vi "DOOR_ASSIGN.vi"(8 "error In":errorcluster) -> (0 "error out":errorcluster)   [LabVIEW 2017]
uses:
  Controls/Ass. Loop Control.ctl
  <vilib>/Utility/error.llb/DialogType.ctl
  <vilib>/Utility/file.llb/Read Delimited Spreadsheet (string).vi
  <vilib>/Utility/file.llb/Write Delimited Spreadsheet (string).vi
  <vilib>/Utility/config.llb/NI_LVConfig.lvlib
panel:
  in  "REMOVE PART":bool
  in  "ADD PART":bool
  in  "LIST OF PARTS":string(combo)
  in  "DOORS":string(combo)
  in  "DOORS":enum32{"ADD PARTS", "Page 1", "Page 2"}(tab)
  in  "ADDED PART LIST":string(combo)
  in  "REMOVE PART FROM LIST":bool
  in  "ADD PART IN LIST":bool
  in  "NEW PARTS BARCODE":string
  out "DOOR 1":string[](array[string])
  out "DOOR 2":string[](array[string])
  out "DOOR 3":string[](array[string])
  out "DOOR 4":string[](array[string])
  out "DOOR 5":string[](array[string])
  out "DOOR 16":string[](array[string])
  out "DOOR 11":string[](array[string])
  out "DOOR 12":string[](array[string])
  out "DOOR 13":string[](array[string])
  out "DOOR 14":string[](array[string])
  out "DOOR 15":string[](array[string])
  out "USER:-":string
  in  "Stop":bool
  out "DATE/TIME":string
  out "Screen Name":string
  # "Nm"
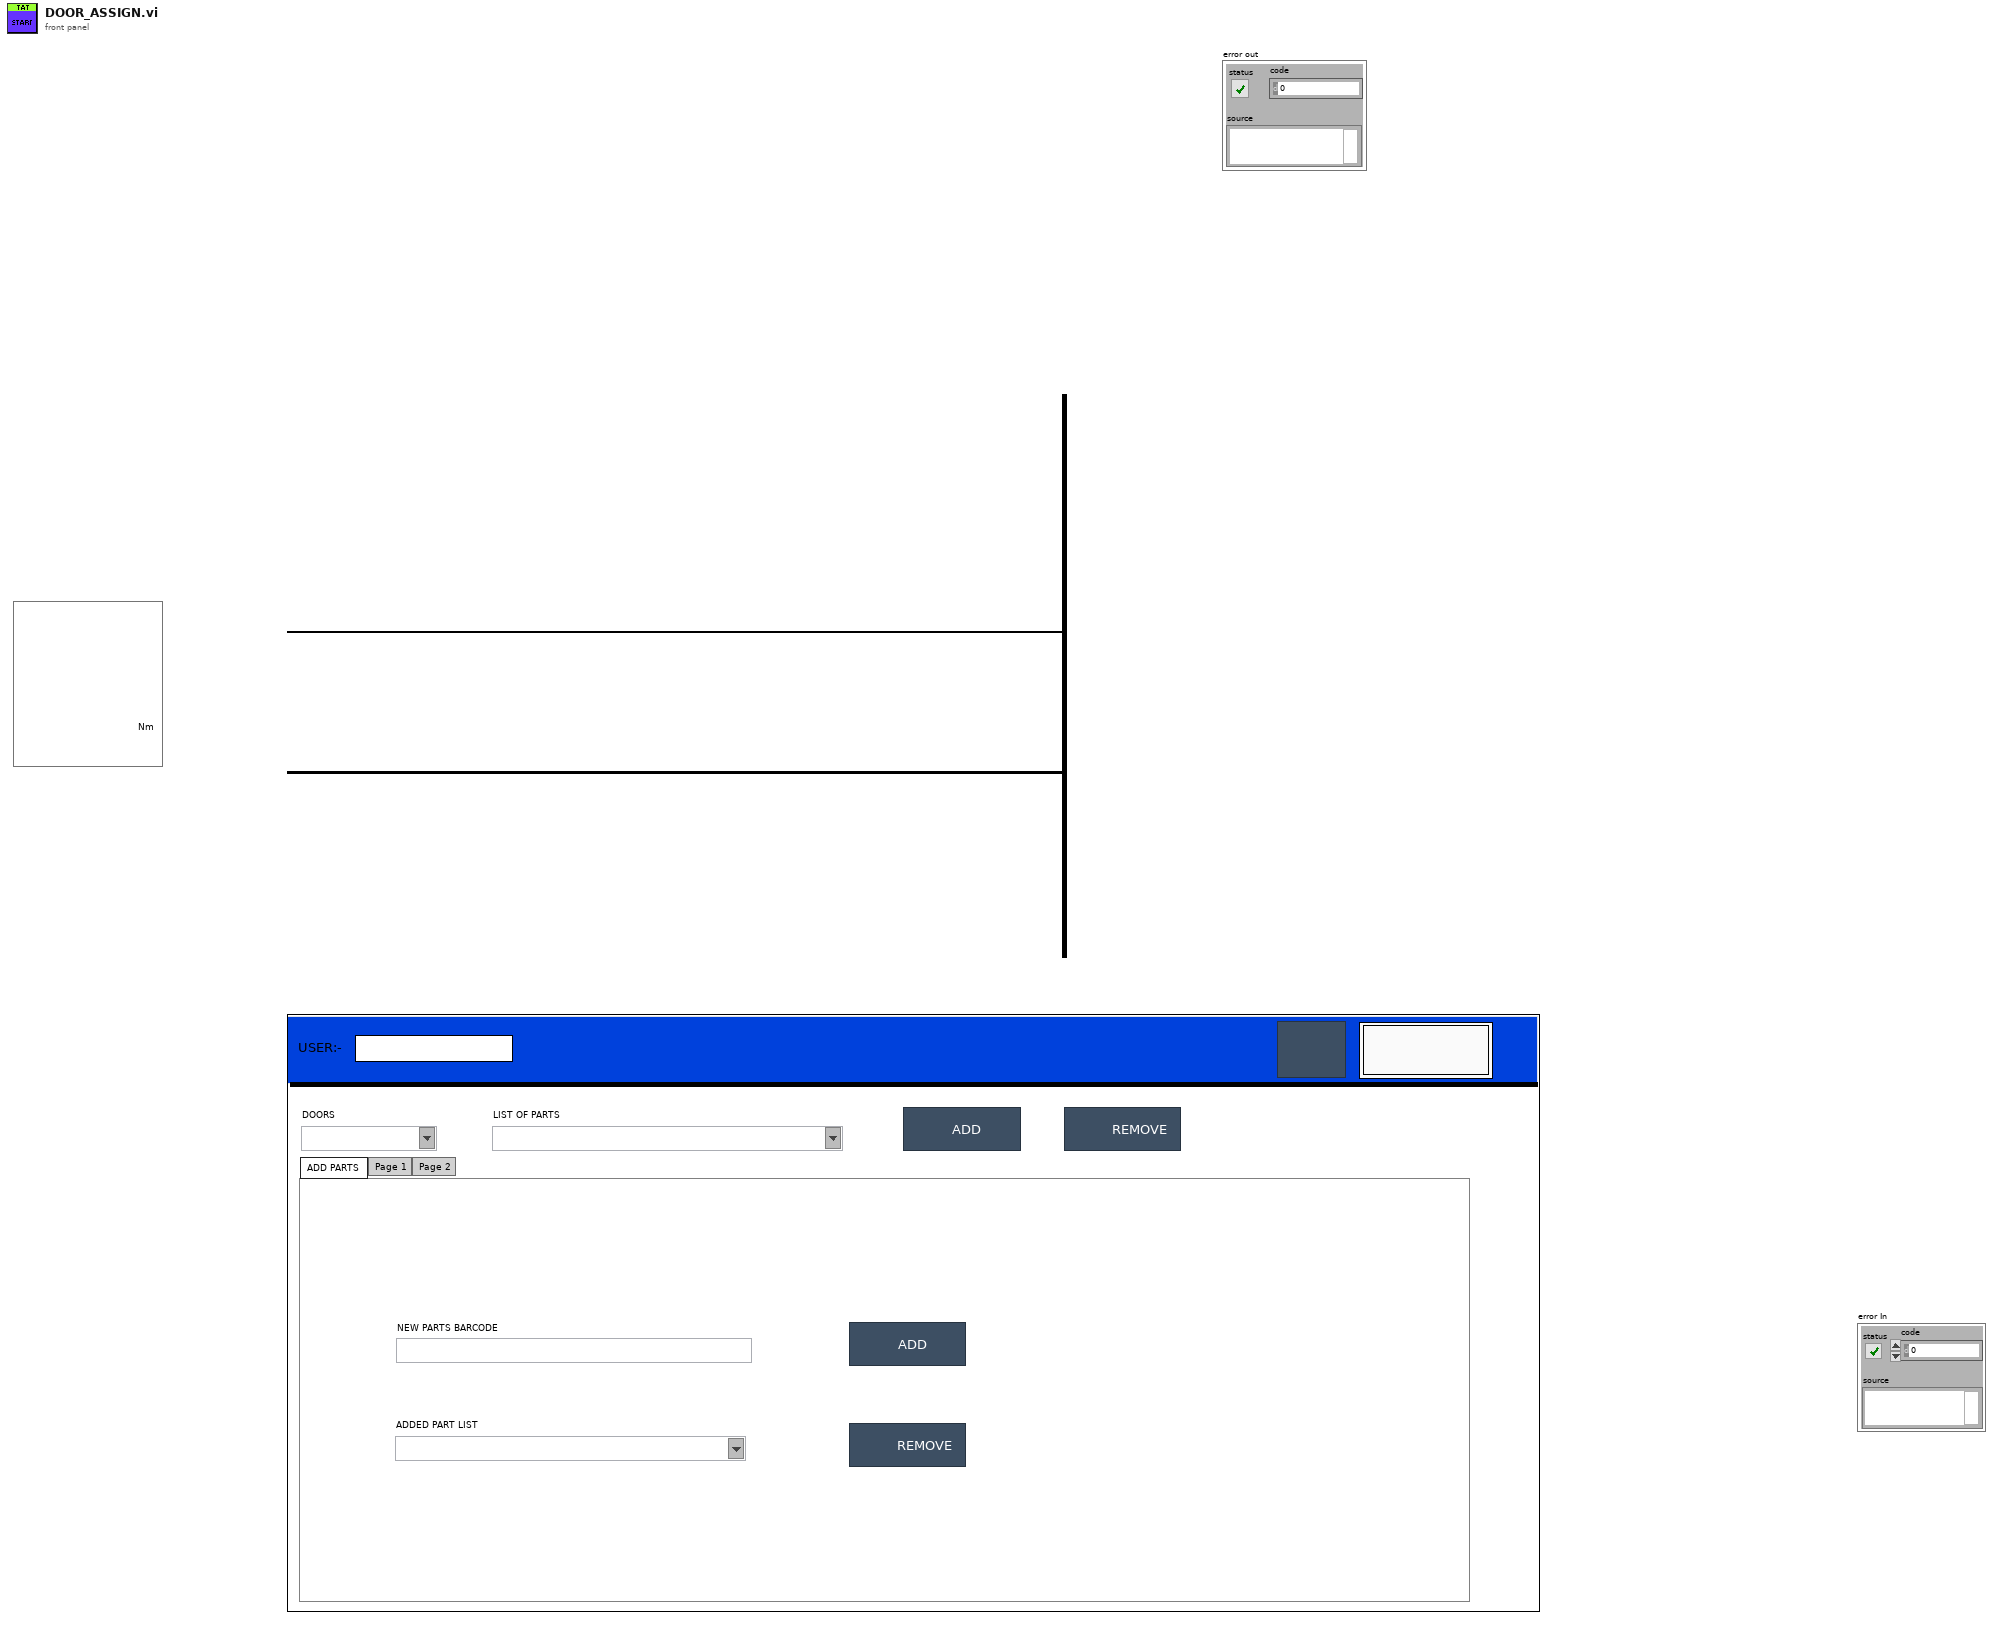
[diagram p1: front panel]
types:
  T1 = cluster{"DOOR ASSIGN":path, "PART LIST":path, "DOOR PART ASSIGN":cluster{"DOOR 1":cluster{"DOOR 1":string[]}, "DOOR 2":cluster{"DOOR 2":string[]}, "DOOR 3":cluster{"DOOR 3":string[]}, "DOOR 4":cluster{"DOOR 4":string[]}, "DOOR 5":cluster{"DOOR 5":string[]}, "DOOR 11":cluster{"DOOR 11":string[]}, "DOOR 12":cluster{"DOOR 12":string[]}, "DOOR 13":cluster{"DOOR 13":string[]}, "DOOR 14":cluster{"DOOR 14":string[]}, "DOOR 15":cluster{"DOOR 15":string[]}, "DOOR 16":cluster{"DOOR 16":string[]}}}
  T2 = typedef "DialogType.ctl" = u16
  T3 = typedef "Ass. Loop Control.ctl" = enum16{"Package_Qty_Count", "GENERATE_QR_PRNT", "Cluster_update", "Waiting_for_scan", "barcode CHECK", "Int", "SaveReport ", "Barcode Print", "Start Cycle", "Wait", "Cycle End", "Stop"}
  T4 = enum32{"invalid app kind", "Development System", "Run Time System", "Student Edition", "Embedded LabVIEW", "Evaluation", "Custom"}
  T5 = cluster{"DOOR 1":string[], "DOOR 2":string[], "DOOR 3":string[], "DOOR 4":string[], "DOOR 5":string[], "DOOR 11":string[], "DOOR 12":string[], "DOOR 13":string[], "DOOR 14":string[], "DOOR 15":string[], "DOOR 16":string[]}
  T6 = typedef "LVComboBoxStrsAndValuesArrayTypeDef.ctl" = cluster{"String":string, "Value":string}[]
  T7 = typedef "NI_LVConfig.lvlib/Config Data RefNum.ctl" = refnum<k1>
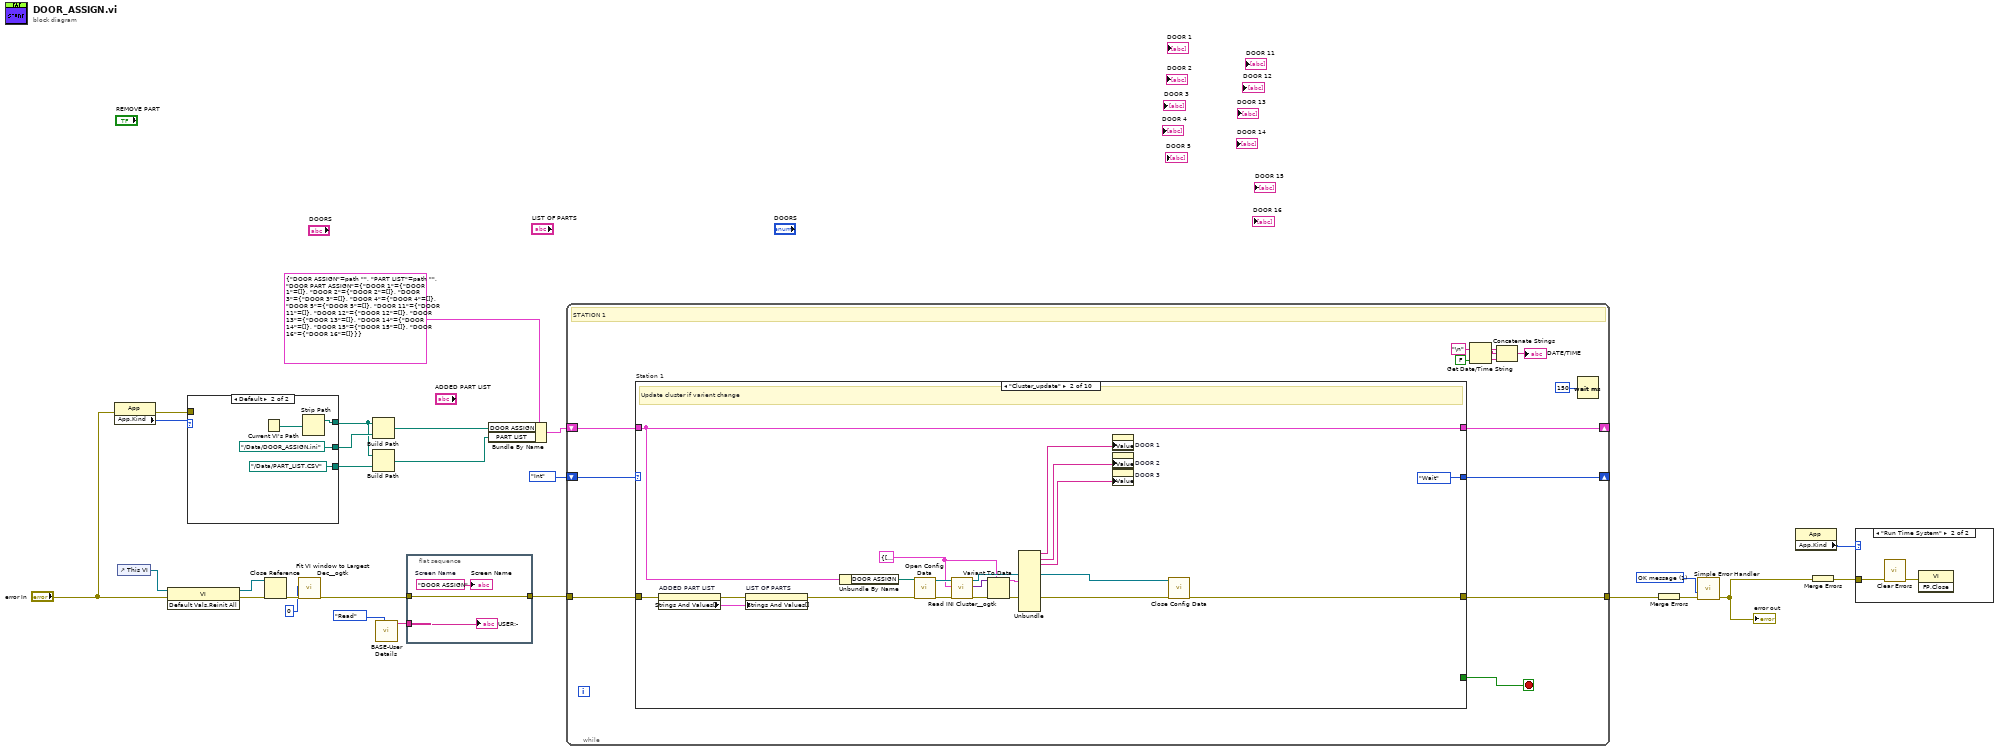
[diagram p0: block diagram]
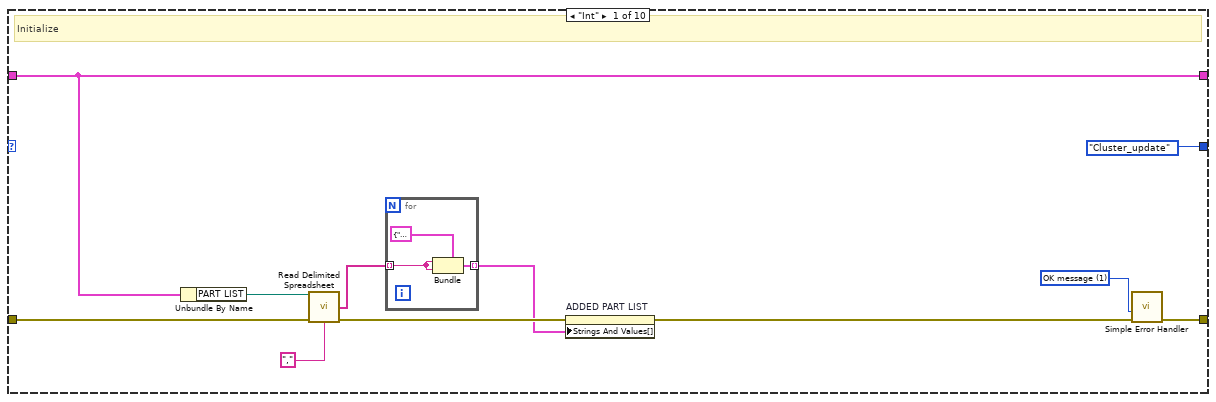
[diagram p3: hidden frame]
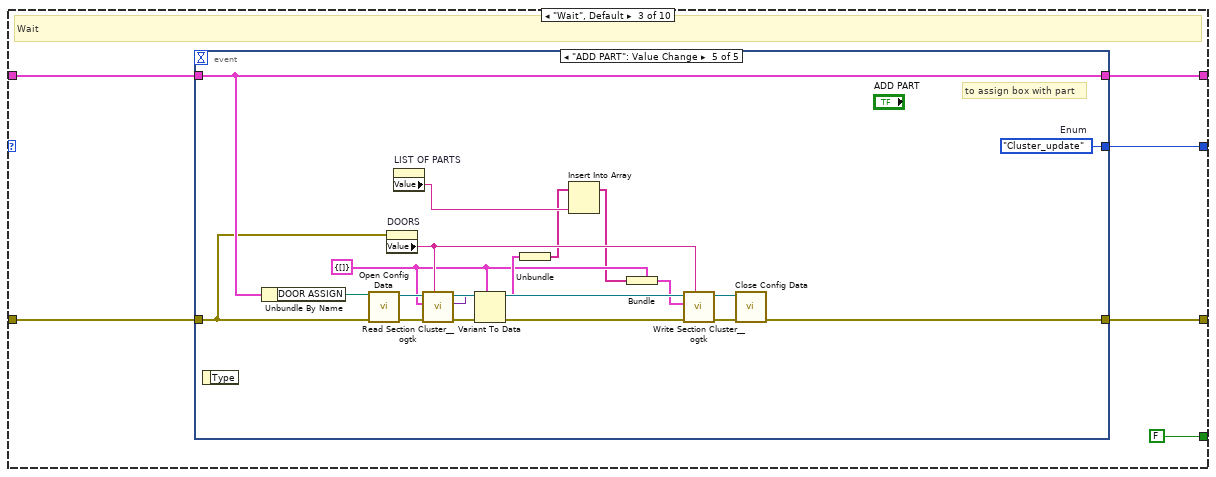
[diagram p4: hidden frame]
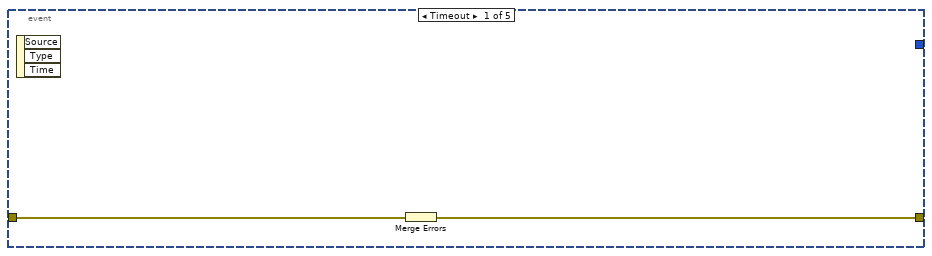
[diagram p5: hidden frame]
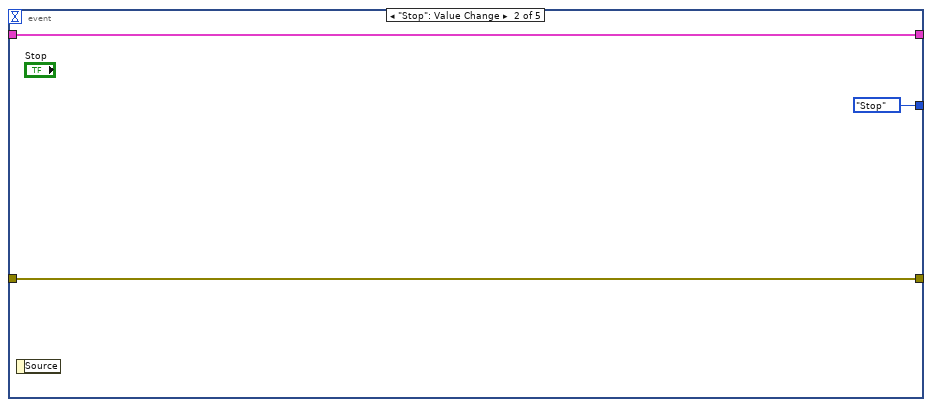
[diagram p6: hidden frame]
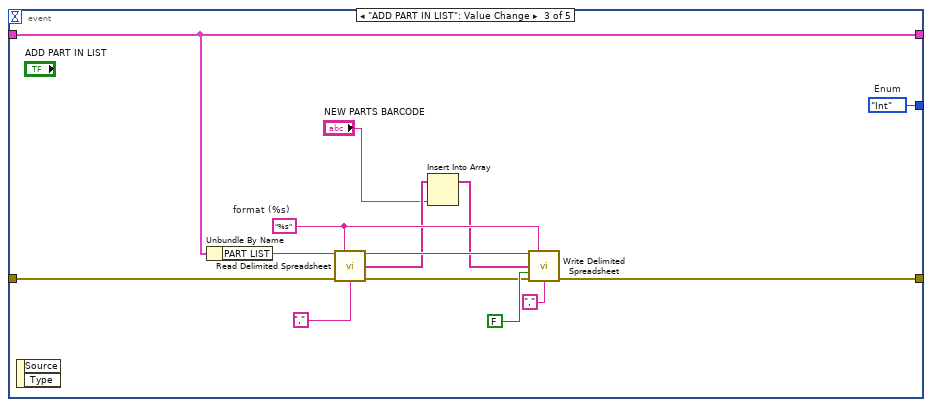
[diagram p7: hidden frame]
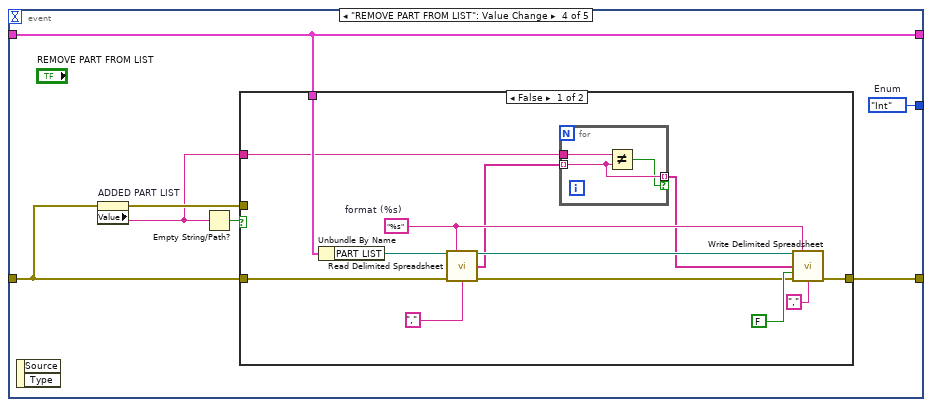
[diagram p8: hidden frame]
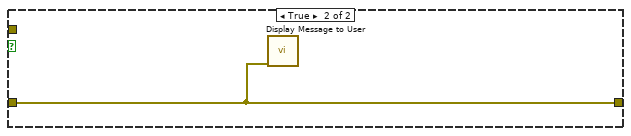
[diagram p9: hidden frame]
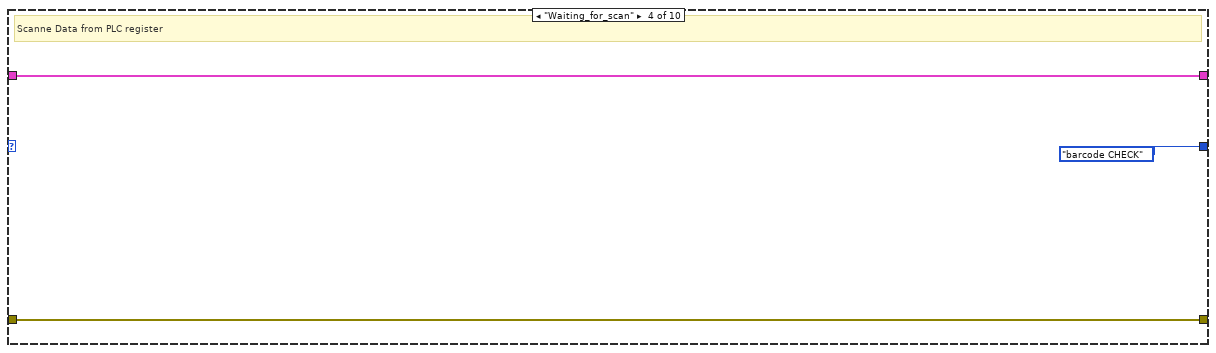
[diagram p10: hidden frame]
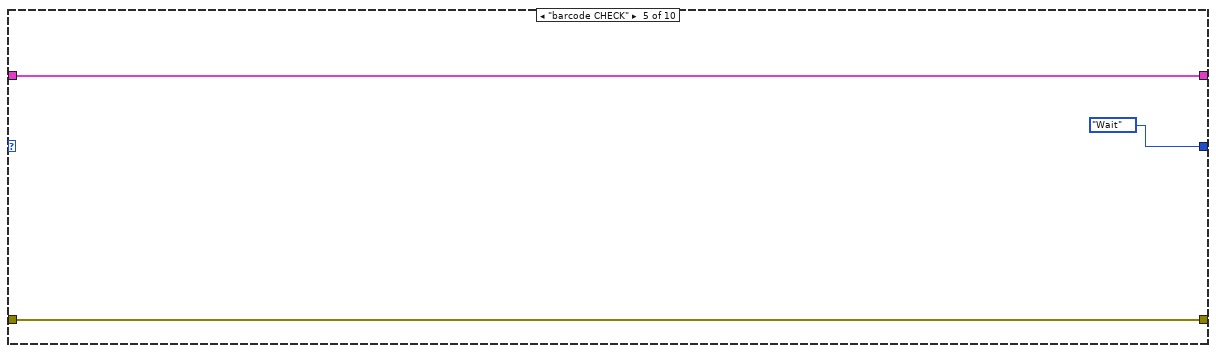
[diagram p11: hidden frame]
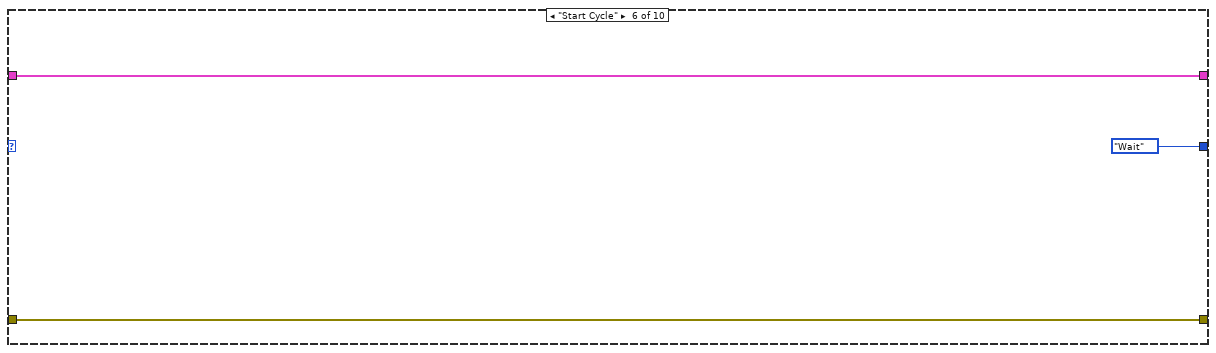
[diagram p12: hidden frame]
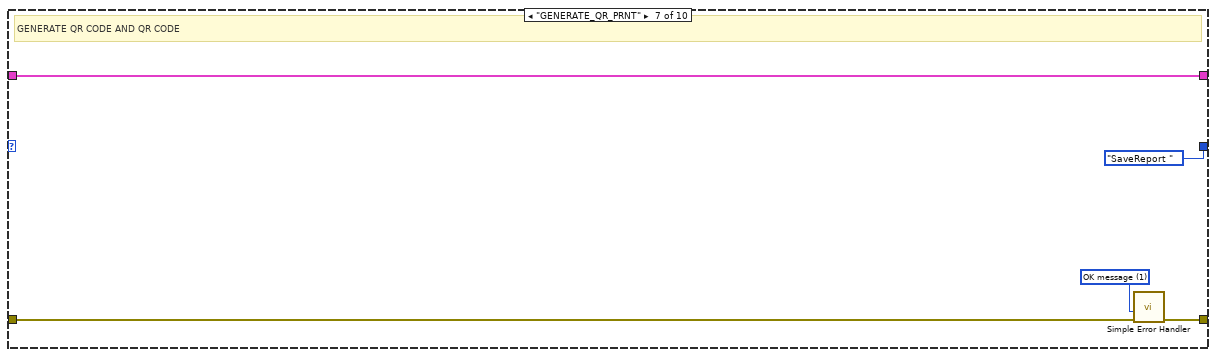
[diagram p13: hidden frame]
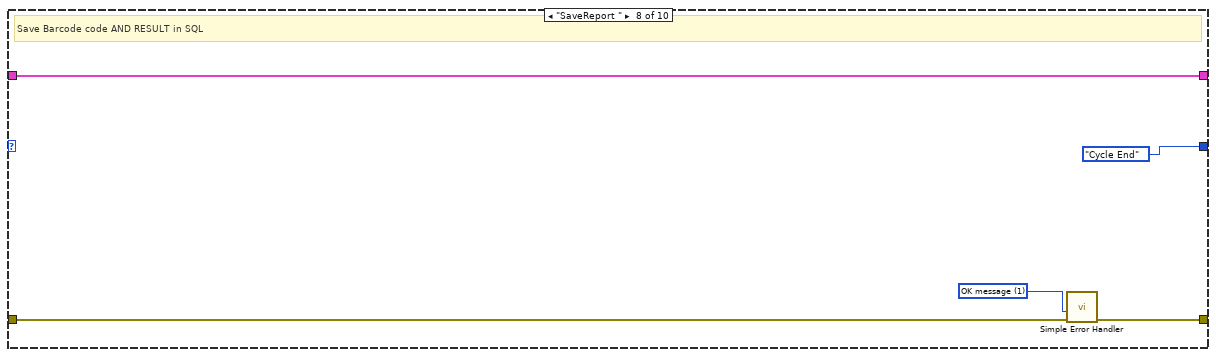
[diagram p14: hidden frame]
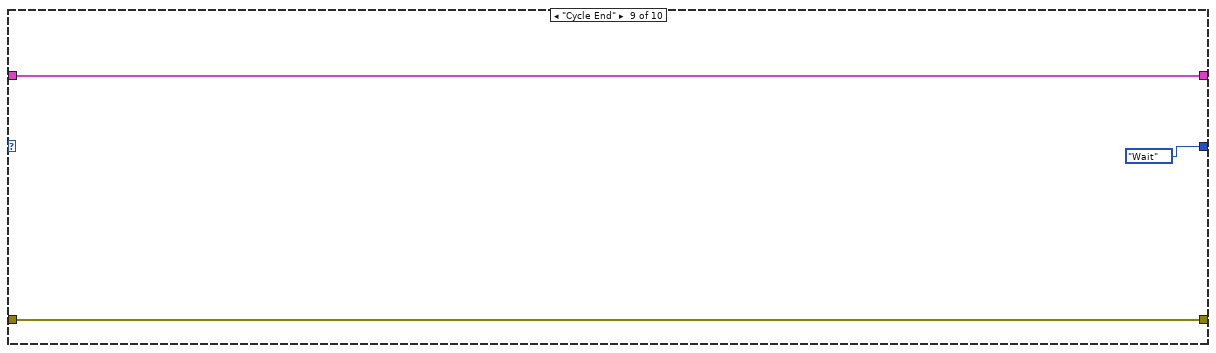
[diagram p15: hidden frame]
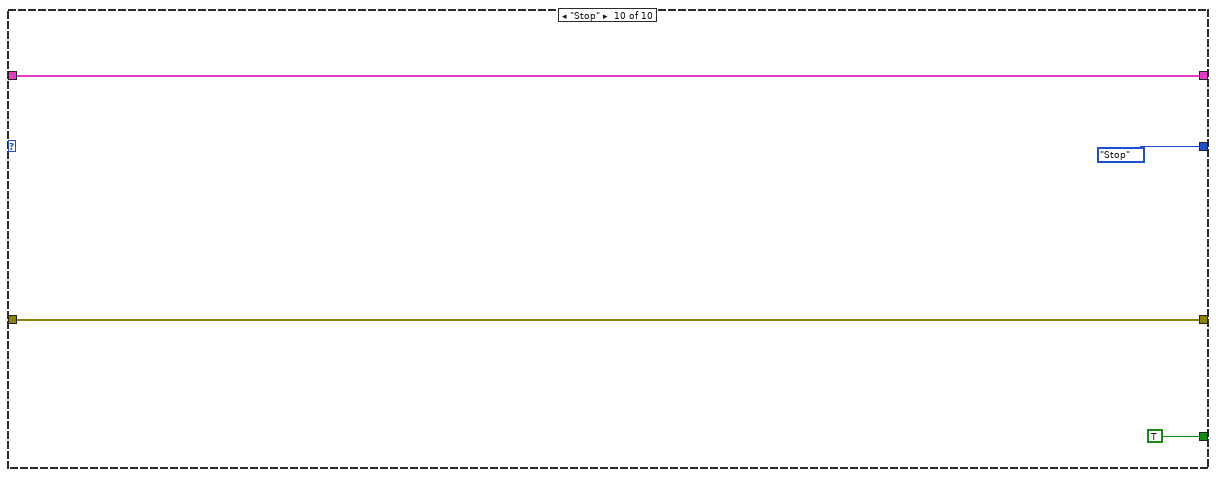
[diagram p16: hidden frame]
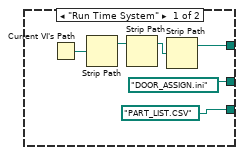
[diagram p17: hidden frame]
diagram:
  w17 = T2 1 items=["no dialog", "OK message", "continue or stop message", "OK message + warnings", "continue/stop + warnings"] ("type of dialog (OK msg:1)")
  n1 = property class="App"(error in="error In") -> (error out=w13:errorcluster, "App.Kind"=w15:T4)  [unwired: 1 in, 1 out]
  n2 = control-ref of="This VI"() -> (w26:refnum<vi>)
  n3 = invoke class="VI" method="Default Vals.Reinit All"(reference=w26, error in="error In") -> (reference out=w24:refnum<vi>, error out=w25:errorcluster)  [unwired: 1 in, 1 out]
  n4 = case shown="Default" w15 {
    tunnel: [path "DOOR_ASSIGN.ini" ("path") path "../Data/DOOR_ASSIGN.ini" ("path")] -> w14
    tunnel: [w28 w34] -> w3
    tunnel: w13 -> [_ _]
    tunnel: [path "PART_LIST.CSV" ("path") path "../Data/PART_LIST.CSV" ("path")] -> w2
    frame "Run Time System" {
      n5 = Current VI's Path() -> (path=w31:path)
      n6 = Strip Path(path=w31) -> (stripped path=w30:path)  [unwired: 1 out]
      n7 = Strip Path(path=w30) -> (stripped path=w29:path)  [unwired: 1 out]
      n8 = Strip Path(path=w29) -> (stripped path=w28:path)  [unwired: 1 out]
    }
    frame Default {
      n9 = Current VI's Path() -> (path=w35:path)
      n10 = Strip Path(path=w35) -> (stripped path=w34:path)  [unwired: 1 out]
    }
  }
  n11 = Close Reference(reference=w24, error in (no error)=w25) -> (error out=w23:errorcluster)
  n12 = call <userlib>:"Fit VI window to Largest Dec__ogtk.vi"("error in (no error)"=w23, "border spacing (2 px)"=0) -> ("error out"=w11:errorcluster)  [unwired: 4 in, 1 out]
  n13 = Build Path(base path=w3, name or relative path=w14) -> (appended path=w4:path)
  n14 = Build Path(base path=w3, name or relative path=w2) -> (appended path=w1:path)
  n15 = call "BASE-User Details.vi"("Enum"=enum16{"Read", "Write"}."Read") -> ("User Name Out"=w18:string)  [unwired: 9 in, 1 out]
  n16 = flat-sequence {
    tunnel: [w39] -> w7
    tunnel: w11 -> [w39]
    tunnel: w18 -> [w38]
    frame #0 {
      w37 = "DOOR ASSIGN"  # Screen Name
      "USER:-" <- w38
      "Screen Name" <- w37
    }
  }
  n17 = Bundle By Name(cluster=T1 {"DOOR ASSIGN"=path "", "PART LIST"=path "", "DOOR PART ASSIGN"={"DOOR 1"={"DOOR 1"=[]}, "DOOR 2"={"DOOR 2"=[]}, "DOOR 3"={"DOOR 3"=[]}, "DOOR 4"={"DOOR 4"=[]}, "DOOR 5"={"DOOR 5"=[]}, "DOOR 11"={"DOOR 11"=[]}, "DOOR 12"={"DOOR 12"=[]}, "DOOR 13"={"DOOR 13"=[]}, "DOOR 14"={"DOOR 14"=[]}, "DOOR 15"={"DOOR 15"=[]}, "DOOR 16"={"DOOR 16"=[]}}}, "DOOR ASSIGN"=w4, "PART LIST"=w1) -> (w5:T1)
  n18 = while {
    tunnel: w7 -> [w42]
    shift-right: [w43] -> _
    shift-left: Ass._Loop_Control."Int" ("Enum") -> [w52]
    tunnel: [w50] -> w21
    shift-right: [w40] -> _
    shift-left: w5 -> [w41]
    stop <- w44 stop-if-true
    # "STATION 1"
    n19 = case "Station 1" shown="\"Cluster_update\"" w52 {
      tunnel: [Ass._Loop_Control."Cluster_update" ("Enum") Ass._Loop_Control."Wait" ("Enum") w88 Ass._Loop_Control."barcode CHECK" ("Enum") Ass._Loop_Control."Wait" ("Enum") Ass._Loop_Control."Wait" ("Enum") Ass._Loop_Control."SaveReport " ("Enum") Ass._Loop_Control."Cycle End" ("Enum") Ass._Loop_Control."Wait" ("Enum") Ass._Loop_Control."Stop" ("Enum")] -> w43
      tunnel: [_ _ FALSE _ _ _ _ _ _ TRUE] -> w44
      tunnel: [w61 w71 w89 w156 w159 w162 w167 w171 w175 w178] -> w50
      tunnel: w42 -> [w57 w82 w90 w156 w159 w162 w165 w170 w175 w178]
      tunnel: w41 -> [w59 w73 w86 w155 w158 w161 w164 w169 w174 w177]
      tunnel: [w59 w73 w87 w155 w158 w161 w164 w169 w174 w177] -> w40
      frame "Int" {
        w62 = T2 1 items=["no dialog", "OK message", "continue or stop message", "OK message + warnings", "continue/stop + warnings"] ("type of dialog (OK msg:1)")
        # "Initialize"
        n20 = Unbundle By Name(w59) -> ("PART LIST"=w58:path)
        n21 = call-poly <vilib>:"Read Delimited Spreadsheet.vi"("file path (dialog if empty)"=w58, "error in (no error)"=w57, "delimiter (\\t)"="," ("format (%s)")) -> ("first row"=w54:string[], "error out"=w56:errorcluster)  [unwired: 7 in, 4 out]
        n22 = for {
          tunnel: w54 -> [w65] mode=indexing
          tunnel: [w64] -> w53 mode=indexing
          n23 = Bundle(cluster=cluster{"String":string, "Value":string} {"String"="", "Value"=""}, "String"=w65, "Value"=w65) -> (w64:cluster{"String":string, "Value":string})
        }
        n24 = property on="ADDED PART LIST" class="CmbBox"(error in=w56, "Strings And Values[]"=w53) -> (error out=w60:errorcluster)  [unwired: 1 in, 1 out]
        n25 = call <vilib>:"Simple Error Handler.vi"("type of dialog (OK msg:1)"=w62, "error in (no error)"=w60) -> ("error out"=w61:errorcluster)  [unwired: 3 in, 4 out]
      }
      frame "Cluster_update" {
        w69 = T5 {"DOOR 1"=[], "DOOR 2"=[], "DOOR 3"=[], "DOOR 4"=[], "DOOR 5"=[], "DOOR 11"=[], "DOOR 12"=[], "DOOR 13"=[], "DOOR 14"=[], "DOOR 15"=[], "DOOR 16"=[]}
        # "Update cluster if varient change"
        n26 = property on="ADDED PART LIST" class="CmbBox"(error in=w82) -> (error out=w83:errorcluster, "Strings And Values[]"=w84:T6)  [unwired: 1 in, 1 out]
        n27 = property on="LIST OF PARTS" class="CmbBox"(error in=w83, "Strings And Values[]"=w84) -> (error out=w72:errorcluster)  [unwired: 1 in, 1 out]
        n28 = Unbundle By Name(w73) -> ("DOOR ASSIGN"=w81:path)
        n29 = call <vilib>:"Open Config Data.vi"("error in (no error)"=w72, "configuration file path"=w81) -> ("error out"=w80:errorcluster, "refnum"=w78:T7)  [unwired: 7 in, 1 out]
        n30 = call <userlib>:"Read INI Cluster__ogtk.vi"("error in (no error)"=w80, "INI Fomatted Cluster Type"=w69, "refnum"=w78) -> ("error out"=w76:errorcluster, "INI Fomatted Cluster"=w77:variant, "dup refnum"=w79:T7)  [unwired: 4 in, 2 out]
        n31 = Variant To Data(error in=w76, type=w69, Variant=w77) -> (data=w74:T5, error out=w75:errorcluster)
        n32 = Unbundle(w74) -> ("DOOR 1"=w70:string[], "DOOR 2"=w68:string[], "DOOR 3"=w67:string[])  [unwired: 8 out]
        n33 = property on="DOOR 1" class="Arr (strict)"("Value"=w70) -> ()  [unwired: 2 in, 2 out]
        n34 = property on="DOOR 2" class="Arr (strict)"("Value"=w68) -> ()  [unwired: 2 in, 2 out]
        n35 = property on="DOOR 3" class="Arr (strict)"("Value"=w67) -> ()  [unwired: 2 in, 2 out]
        n36 = call <vilib>:"Close Config Data.vi"("error in (no error)"=w75, "refnum"=w79) -> ("error out"=w71:errorcluster)  [unwired: 8 in, 1 out]
      }
      frame "Wait", Default {
        # "Wait"
        n37 = event shown="[4] \"ADD PART\": Value Change" {
          selector: _ -> [_ _ _ _ _]
          dyn-events: _ -> [_ _ _ _ _]
          timeout: _ -> [_ _ _ _ _]
          tunnel: w90 -> [w93 w95 w104 w114 w148]
          tunnel: [w92 w95 w103 w116 w152] -> w89
          tunnel: [_ Ass._Loop_Control."Stop" ("Enum") w97 w115 w151] -> w88
          tunnel: [_ w94 w108 w117 w150] -> w87
          tunnel: w86 -> [_ w94 w108 w117 w150]
          event Timeout {
            n38 = event-data() -> ()  [unwired: 1 in, 3 out]
            n39 = Merge Errors(w93) -> (w92:errorcluster)
          }
          event "Stop": Value Change {
            n40 = event-data() -> ()  [unwired: 1 in, 1 out]
          }
          event "ADD PART IN LIST": Value Change {
            w97 = Ass._Loop_Control."Int"  # Enum
            w101 = "%s"  # format (%s)
            n41 = event-data() -> ()  [unwired: 1 in, 2 out]
            n42 = Unbundle By Name(w108) -> ("PART LIST"=w110:path)
            n43 = call-poly <vilib>:"Read Delimited Spreadsheet.vi"("file path (dialog if empty)"=w110, "format (%s)"=w101, "error in (no error)"=w104, "delimiter (\\t)"="," ("format (%s)")) -> ("new file path (Not A Path if cancelled)"=w106:path, "first row"=w100:string[], "error out"=w105:errorcluster)  [unwired: 6 in, 3 out]
            n44 = Insert Into Array(array=w100, new element="NEW PARTS BARCODE") -> (w98:string[])  [unwired: 1 in]
            n45 = call-poly <vilib>:"Write Delimited Spreadsheet.vi"("file path (dialog if empty)"=w106, "format (%s)"=w101, "1D data"=w98, "append to file? (new file:F)"=FALSE, "error in (no error)"=w105, "delimiter (\\t)"="," ("format (%s)")) -> ("error out"=w103:errorcluster)  [unwired: 8 in, 1 out]
          }
          event "REMOVE PART FROM LIST": Value Change {
            w115 = Ass._Loop_Control."Int"  # Enum
            n46 = event-data() -> ()  [unwired: 1 in, 2 out]
            n47 = property on="ADDED PART LIST" class="CmbBox"(error in=w114) -> (error out=w112:errorcluster, "Value"=w111:string)  [unwired: 1 in, 1 out]
            n48 = Empty String/Path?(string/path=w111) -> (empty?=w113:bool)
            n49 = case shown="False" w113 {
              tunnel: w117 -> [w128 _]
              tunnel: [w124 w134] -> w116
              tunnel: w114 -> [w121 w134]
              tunnel: w112 -> [_ _]
              tunnel: w111 -> [w119 _]
              frame False {
                w122 = "%s"  # format (%s)
                n50 = Unbundle By Name(w128) -> ("PART LIST"=w130:path)
                n51 = call-poly <vilib>:"Read Delimited Spreadsheet.vi"("file path (dialog if empty)"=w130, "format (%s)"=w122, "error in (no error)"=w121, "delimiter (\\t)"="," ("format (%s)")) -> ("new file path (Not A Path if cancelled)"=w126:path, "first row"=w120:string[], "error out"=w125:errorcluster)  [unwired: 6 in, 3 out]
                n52 = for {
                  tunnel: w120 -> [w132] mode=indexing
                  tunnel: w119 -> [w133]
                  tunnel: [w132] -> w118 mode=indexing if=w131
                  n53 = Not Equal?(x=w133, y=w132) -> (x != y?=w131:bool)
                }
                n54 = call-poly <vilib>:"Write Delimited Spreadsheet.vi"("file path (dialog if empty)"=w126, "format (%s)"=w122, "1D data"=w118, "append to file? (new file:F)"=FALSE, "error in (no error)"=w125, "delimiter (\\t)"="," ("format (%s)")) -> ("error out"=w124:errorcluster)  [unwired: 8 in, 1 out]
              }
              frame True {
                n55 = call "Display Message to User"("error in (no error)"=w134) -> ()  [unwired: 9 in, 2 out]
              }
            }
          }
          event "ADD PART": Value Change {
            w137 = cluster{"BARCODE":string[]} {"BARCODE"=[]}
            w151 = Ass._Loop_Control."Cluster_update"  # Enum
            # "to assign box with part"
            n56 = event-data() -> ()  [unwired: 1 in, 1 out]
            n57 = Unbundle By Name(w150) -> ("DOOR ASSIGN"=w149:path)
            n58 = call <vilib>:"Open Config Data.vi"("error in (no error)"=w148, "configuration file path"=w149) -> ("error out"=w147:errorcluster, "refnum"=w145:T7)  [unwired: 7 in, 1 out]
            n59 = property on="DOORS" class="CmbBox"(error in=w148) -> ("Value"=w144:string)  [unwired: 1 in, 2 out]
            n60 = property on="LIST OF PARTS" class="CmbBox"() -> ("Value"=w140:string)  [unwired: 2 in, 2 out]
            n61 = call <userlib>:"Read Section Cluster__ogtk.vi"("section (optional)"=w144, "error in (no error)"=w147, "Section Formatted Cluster Type"=w137, "refnum"=w145) -> ("error out"=w142:errorcluster, "Section Formatted Cluster"=w143:variant, "dup refnum"=w146:T7)  [unwired: 3 in, 2 out]
            n62 = Variant To Data(error in=w142, type=w137, Variant=w143) -> (data=w139:cluster{"BARCODE":string[]}, error out=w141:errorcluster)
            n63 = Unbundle(w139) -> ("BARCODE"=w138:string[])
            n64 = Insert Into Array(array=w138, new element=w140) -> (w136:string[])  [unwired: 1 in]
            n65 = Bundle(cluster=w137, "BARCODE"=w136) -> (w135:cluster{"BARCODE":string[]})
            n66 = call <userlib>:"Write Section Cluster__ogtk.vi"("section (optional)"=w144, "error in (no error)"=w141, "Section Formatted Cluster"=w135, "refnum"=w146) -> ("error out"=w153:errorcluster, "dup refnum"=w154:T7)  [unwired: 6 in]
            n67 = call <vilib>:"Close Config Data.vi"("error in (no error)"=w153, "refnum"=w154) -> ("error out"=w152:errorcluster)  [unwired: 8 in, 1 out]
          }
        }
      }
      frame "Waiting_for_scan" {
        # "Scanne Data from PLC register"
      }
      frame "barcode CHECK" {
      }
      frame "Start Cycle" {
      }
      frame "GENERATE_QR_PRNT" {
        w168 = T2 1 items=["no dialog", "OK message", "continue or stop message", "OK message + warnings", "continue/stop + warnings"] ("type of dialog (OK msg:1)")
        # "GENERATE QR CODE AND QR CODE"
        n68 = call <vilib>:"Simple Error Handler.vi"("type of dialog (OK msg:1)"=w168, "error in (no error)"=w165) -> ("error out"=w167:errorcluster)  [unwired: 3 in, 4 out]
      }
      frame "SaveReport " {
        w172 = T2 1 items=["no dialog", "OK message", "continue or stop message", "OK message + warnings", "continue/stop + warnings"] ("type of dialog (OK msg:1)")
        # "Save Barcode code AND RESULT in SQL"
        n69 = call <vilib>:"Simple Error Handler.vi"("type of dialog (OK msg:1)"=w172, "error in (no error)"=w170) -> ("error out"=w171:errorcluster)  [unwired: 3 in, 4 out]
      }
      frame "Cycle End" {
      }
      frame "Stop" {
      }
    }
    n70 = Get Date/Time String(want seconds? (F)=FALSE) -> (date string=w48:string, time string=w47:string)  [unwired: 2 in]
    n71 = Concatenate Strings(w48, "\n", w47) -> (→"DATE/TIME":string)
    n72 = Wait (ms)(milliseconds to wait=u32 150) -> ()  [unwired: 1 out]
  }
  n73 = Merge Errors(w21) -> (w20:errorcluster)
  n74 = call <vilib>:"Simple Error Handler.vi"("type of dialog (OK msg:1)"=w17, "error in (no error)"=w20) -> ("error out"=w8:errorcluster)  [unwired: 3 in, 4 out]
  "error out" <- w8
  n75 = property class="App"() -> ("App.Kind"=w16:T4)  [unwired: 2 in, 2 out]
  n76 = Merge Errors(w8) -> (w9:errorcluster)
  n77 = case shown="\"Run Time System\"" w16 {
    tunnel: w9 -> [_ w182]
    frame "invalid app kind", Default {
    }
    frame "Run Time System" {
      n78 = call <vilib>:"Clear Errors.vi"("error in (no error)"=w182) -> ("error out"=w181:errorcluster)  [unwired: 5 in, 1 out]
      n79 = invoke class="VI" method="FP.Close"(error in=w181) -> ()  [unwired: 2 in, 3 out]
    }
  }
